vi "Get Trigger Enable Phase.vi"(8 "error in":errorcluster, 11 "FPGA VI Reference In":T1) -> (0 "error out":errorcluster, 2 "phase value":u16, 3 "FPGA VI Reference Out":T1)   [LabVIEW 2011, in "FlexRIO Host Library (User).lvlib"]
uses:
  FlexRIO Host Library (User).lvlib
  <vilib>/rvi/interface/nirviReadWriteControl/nirviReadWriteControl.xnode
  Session/FPGA Session Ref.ctl
  Zeiss Acquisition Demo/FPGA Bitfiles/FlexRIODigitizer_FPGABoard_Acquire_Rev2.lvbitx
  <vilib>/rvi/errors/niLvFpgaMergeErrorWithErrorCode.vi
  <vilib>/rvi/errors/niLvFpgaAdjustHostInterfaceError.vi
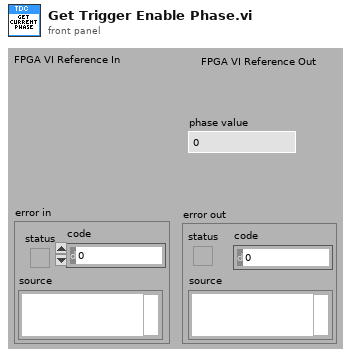
[diagram p1: front panel]
types:
  T1 = typedef "FlexRIO Host.lvlib/FPGA Session Ref.ctl" = refnum<k20>
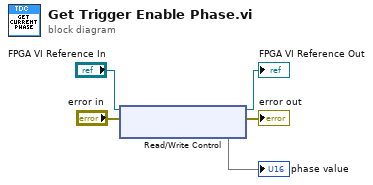
[diagram p0: block diagram]
diagram:
  n1 = xnode "Read/Write Control"("FPGA VI Reference In"="FPGA VI Reference In", "error in"="error in") -> ("FPGA VI Reference Out"=→"FPGA VI Reference Out":T1, "error out"=→"error out":errorcluster, "trigger enable adjust"=→"phase value")
